vi "Vision Processing.vi"(4 "error in (no error)":errorcluster, 6 "CameraDevRef":T1) -> ()   [LabVIEW 2011]
uses:
  <vilib>/Rock Robotics/WPI/Camera/WPI_CameraDevRef.ctl
  Robot Global Data.vi
  <vilib>/vision/NI_Vision_Development_Module.lvlib
panel:
  in  "Run Calculations":bool
  out "Raw Turret":dbl
  out "Target X Coord":dbl
  out "Target Distance":dbl
  out "Target Y Coord":dbl
  out "Distance Array":dbl[](array[numeric])
  in  "Scaler":dbl=0.85
  in  "Lower Speed Limit":dbl=0.05
  out "Number of Rectangles Visible":dbl
  out "Y Position Array":dbl[](array[numeric])
  out "X Position Array":dbl[](array[numeric])
  in  "View":bool
  out "Target Info":T2(array[cluster])
  in  "Area Size Limit":i32=444
  in  "Particle Count Limit":i32=8
  in  "Score Limits":T3={"Rect Coverage"=76.0, "Aspect Ratio"=40.0, "X Edge Strength"=40.0, "Y Edge Strength"=60.0}
  in  "Processing":enum32{"Color", "Intensity", "Intensity Open"}(tab)=enum."Intensity Open"
  in  "Luminance":i32=255
  in  "Saturation":i32=255
  in  "Hue":i32(knob)=65 scale=0.0..255.0
  in  "Margins":cluster{"Hue":i32, "Sat":i32, "Lum":i32}={"Hue"=20, "Sat"=27, "Lum"=30} {"Sat" scale=0.0..40.0; "Lum" scale=0.0..40.0; "Hue" scale=0.0..40.0}
  in  "Range":cluster{"Lower value":sgl, "Upper value":sgl}={"Lower value"=150.0, "Upper value"=255.0} {"Lower value" scale=0.0..255.0; "Upper value" scale=0.0..255.0}
  in  "Range":cluster{"Lower value":sgl, "Upper value":sgl}={"Lower value"=123.804344, "Upper value"=255.0} {"Lower value" scale=0.0..255.0; "Upper value" scale=0.0..255.0}
  in  "View":bool
  out "Processed Image":T4(plugin-control)
  out "Original Image":T4(plugin-control)
  # "Instructions:\nProcessing the reflective tape that is illuminated by a ring light can be based\non color or light intensity.\nParticles within the image are scored by rectangle coverage, aspect ratio, and\nfor being hollow with a bold edge. A particle is considered a target if all scores\nare above the score limits. Particles can be annotated -- surrounded by\na rectangle and scores drawn to the left .\nTo control the number of particles being scored, use the count limit and the size\nlimit."
  # "To debug, Enable using the View button.\nFor color processing, you can click in the image to select the color for processing."
  # "Enable by clicking the View button.\nGreen scores are above the limit, orange are below. Inner/outer rect\nindicates all passed."
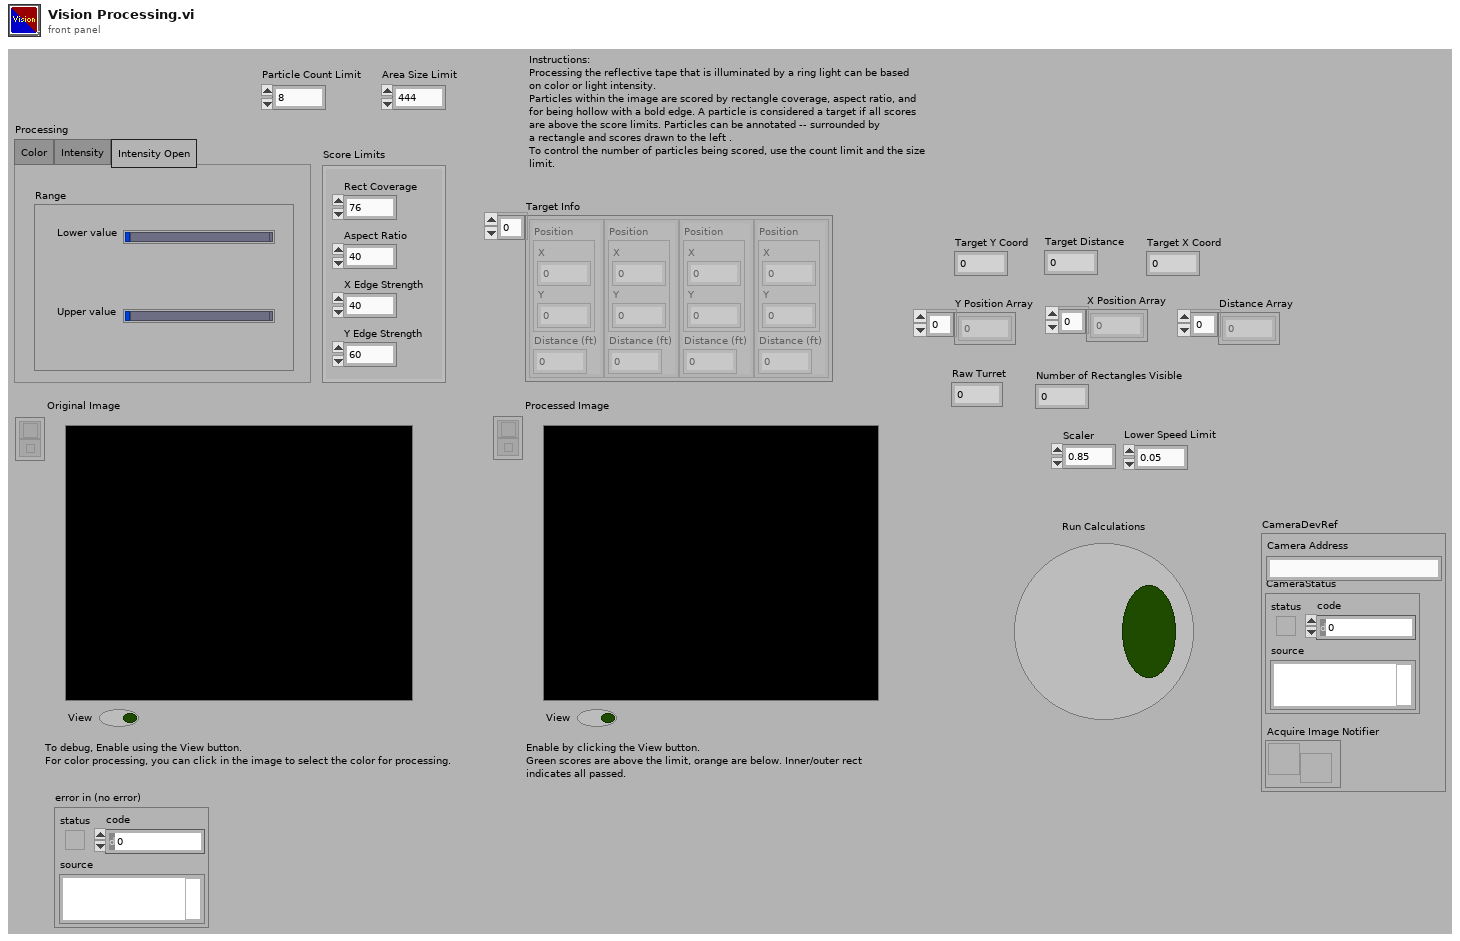
[diagram p1: front panel]
types:
  T1 = typedef "WPI_CameraDevRef.ctl" = cluster{"Camera Address":string, "CameraStatus":errorcluster, "Acquire Image Notifier":refnum<notifier>}
  T2 = cluster{"Position":cluster{"X":dbl, "Y":dbl}, "Distance (ft)":dbl}[]
  T3 = cluster{"Rect Coverage":dbl, "Aspect Ratio":dbl, "X Edge Strength":dbl, "Y Edge Strength":dbl}
  T4 = typedef "IMAQ Image.ctl" = refnum<image>
  T5 = typedef "Image Type" = u32
  T6 = enum32{"AutoM", "Close", "Dilate", "Erode", "Gradient", "Gradient out", "Gradient in", "Hit miss", "Open", "PClose", "POpen", "Thick", "Thin"}
  T7 = typedef "WPI_CameraImageSize.ctl" = enum16{"640x480", "320x240", "160x120"}
  T8 = cluster{"fps":i32, "compression":i32, "Image Size":T7}
  T9 = cluster{cluster{"Left":dbl, "Top":dbl, "Right":dbl, "Bottom":dbl}, dbl[]}[]
  T10 = cluster{"Left":dbl, "Top":dbl, "Right":dbl, "Bottom":dbl}
  T11 = cluster{"Target Center (-1 to 1)":cluster{"X":dbl, "Y":dbl}, "Distance (ft)":dbl}
  T12 = cluster{"Target Center (-1 to 1)":cluster{"X":dbl, "Y":dbl}, "Distance (ft)":dbl}[]
  T13 = typedef "WPI_JoystickDevRef.ctl" = cluster{"Device":T14}
  T14 = typedef "WPI_JoystickDeviceEnum.ctl" = enum16{"USB 1", "USB 2", "USB 3", "USB 4", "Kinect 1", "Kinect 2"}
  T15 = typedef "WPI_JoystickButtonState.ctl" = cluster{"Button 1":bool, "Button 2":bool, "Button 3":bool, "Button 4":bool, "Button 5":bool, "Button 6":bool, "Button 7":bool, "Button 8":bool, "Button 9":bool, "Button 10":bool, "Button 11":bool, "Button 12":bool}
  T16 = cluster{"axis 1 (x)":dbl, "axis 2 (y)":dbl, "axis 3 (throttle)":dbl, "axis 4":dbl, "axis 5":dbl, "axis 6":dbl}
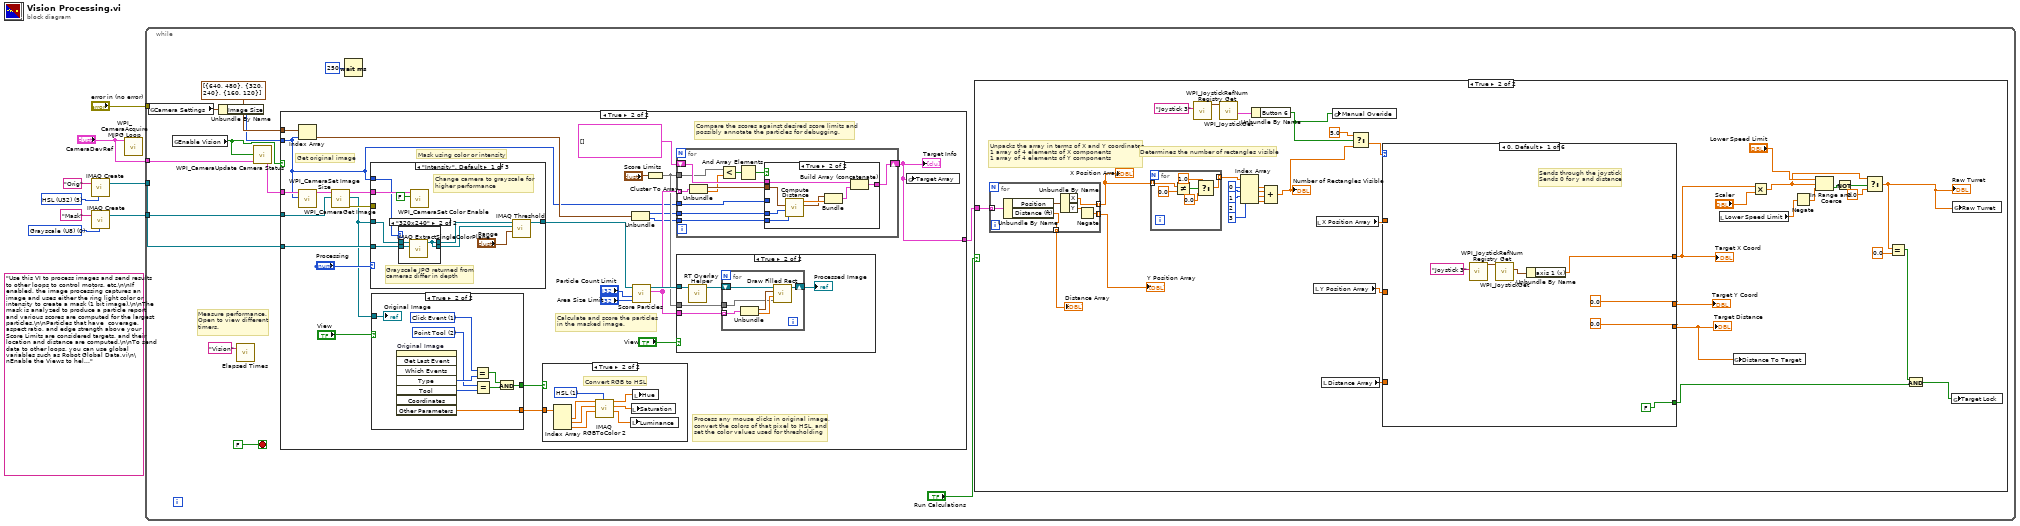
[diagram p0: block diagram]
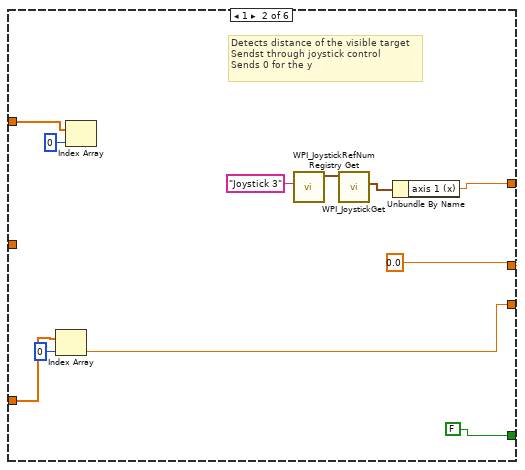
[diagram p3: hidden frame]
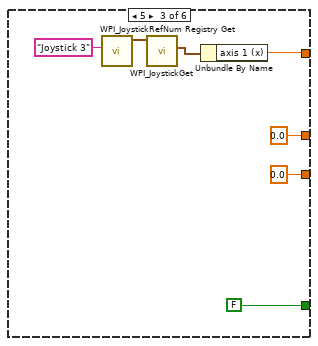
[diagram p4: hidden frame]
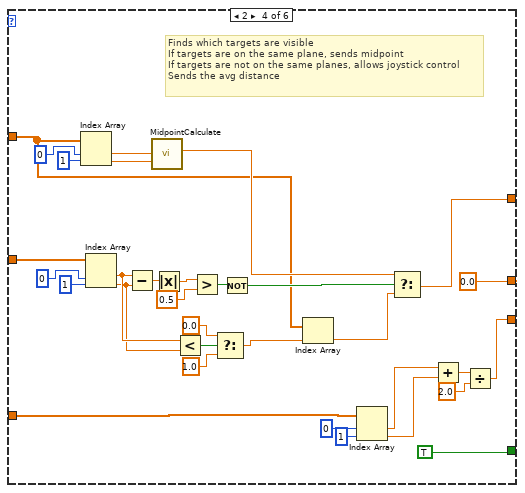
[diagram p5: hidden frame]
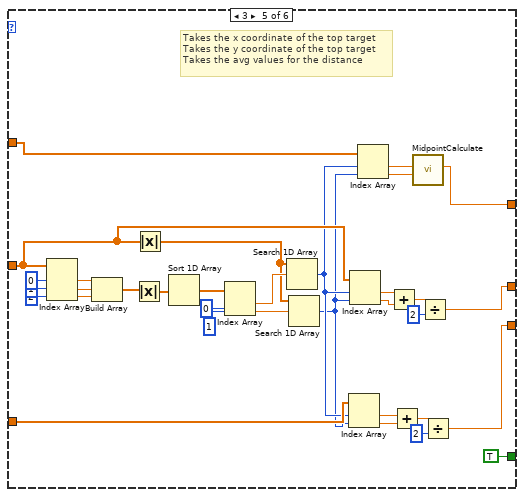
[diagram p6: hidden frame]
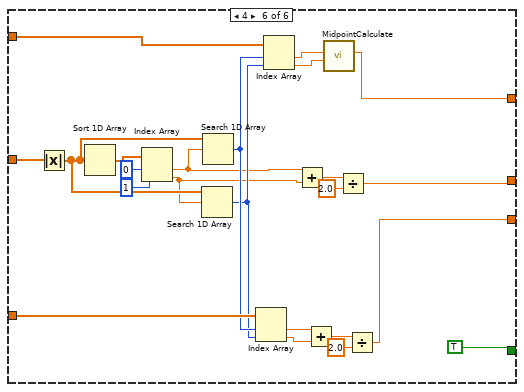
[diagram p7: hidden frame]
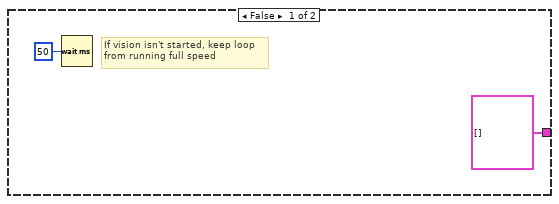
[diagram p8: hidden frame]
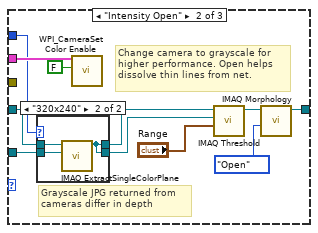
[diagram p11: hidden frame]
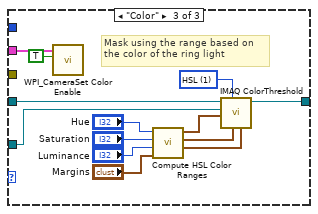
[diagram p13: hidden frame]
diagram:
  w3 = T5 0 items=["Grayscale (U8)", "Grayscale (I16)", "Grayscale (SGL)", "Complex (CSG)", "RGB (U32)", "HSL (U32)", "RGB (U64)", "Grayscale (U16)"] ("Image Type")
  (unwired) "Use this VI to process images and send results to other loops to control motors, etc.\n\nIf enabled, the image processing captures an image and uses either the ring light color or intensity to create a mask (1 bit image).\n\nThe mask is analyzed to produce a particle report and various scores are computed for the largest particles.\n\nParticles that have  coverage, aspect ratio, and edge strength above your Score Limits are considered targets, and their location and distance are computed.\n\nTo send data to other loops, you can use global variables such as Robot Global Data.vi\n\nEnable the Views to help debug color settings. Disable the View to speed up processing."
  w7 = T5 5 items=["Grayscale (U8)", "Grayscale (I16)", "Grayscale (SGL)", "Complex (CSG)", "RGB (U32)", "HSL (U32)", "RGB (U64)", "Grayscale (U16)"] ("Image Type")
  n1 = call "IMAQ Create"("Image Name"="Orig", "Image Type"=w7) -> ("New Image"=w6:T4)  [unwired: 2 in, 2 out]
  n2 = call "IMAQ Create"("Image Name"="Mask", "Image Type"=w3) -> ("New Image"=w1:T4)  [unwired: 2 in, 2 out]
  n3 = call <vilib>:"WPI_CameraAcquire MJPG Loop.vi"("CameraDevRef"="CameraDevRef") -> ()  [unwired: 11 in]
  n4 = while {
    tunnel: w6 -> [w20]
    tunnel: "CameraDevRef" -> [w19]
    tunnel: "error in (no error)" -> [_]
    tunnel: w1 -> [w15]
    stop <- FALSE stop-if-true
    # "Measure performance.\nOpen to view different\ntimers."
    n5 = global read "Robot Global Data.vi" "Camera Settings"() -> (w13:T8)
    n6 = global read "Robot Global Data.vi" "Enable Vision"() -> (w17:bool)
    n7 = Unbundle By Name(w13) -> ("Image Size"=w12:T7)
    n8 = call "Elapsed Times.vi"("Call Name"="Vision") -> ()  [unwired: 2 in, 1 out]
    n9 = call <vilib>:"WPI_CameraUpdate Camera Status.vi"("CameraDevRef In"=w19, "Enable Vision"=w17) -> ("CameraDevRef Out"=w18:T1)  [unwired: 3 in]
    n10 = case shown="True" w17 {
      tunnel: w20 -> [_ w204]
      tunnel: w18 -> [_ w200]
      tunnel: w15 -> [_ w191]
      tunnel: cluster{i32, i32}[] [{640, 480}, {320, 240}, {160, 120}] -> [_ w195]
      tunnel: w12 -> [_ w188]
      tunnel: [T2 [] w189] -> w11
      frame False {
        # "If vision isn't started, keep loop\nfrom running full speed"
        n11 = Wait (ms)(milliseconds to wait=u32 50) -> ()  [unwired: 1 out]
      }
      frame True {
        # "Compare the scores against desired score limits and\npossibly annotate the particles for debugging."
        # "Process any mouse clicks in original image,\nconvert the colors of that pixel to HSL, and\nset the color values used for thresholding"
        # "Calculate and score the particles\nin the masked image."
        # "Mask using color or intensity"
        # "Get original image"
        n12 = call <vilib>:"WPI_CameraSet Image Size.vi"("Image Size"=w188, "CameraDevRef"=w200) -> ("CameraDevRef Out"=w201:T1)  [unwired: 8 in, 1 out]
        n13 = Index Array(array=w195, index=w188) -> (element=w192:cluster{i32, i32})
        n14 = call <vilib>:"WPI_CameraGet Image.vi"("Image"=w204, "CameraDevRef"=w201) -> ("error out"=w202:errorcluster, "Image Out"=w190:T4, "CameraDevRef Out"=w203:T1)  [unwired: 7 in]
        n15 = case shown="\"Intensity\", Default" "Processing" {
          tunnel: w190 -> [w226 w238 w264]
          tunnel: [w229 w243 w263] -> w198
          tunnel: w203 -> [w227 w241 w254]
          tunnel: w202 -> [_ _ _]
          tunnel: w191 -> [w225 w239 w252]
          tunnel: w188 -> [w224 w240 _]
          frame "Intensity", Default {
            # "Grayscale JPG returned from\ncameras differ in depth"
            # "Change camera to grayscale for\nhigher performance"
            n16 = case shown="\"320x240\"" w224 {
              tunnel: w226 -> [w232 w235]
              tunnel: w225 -> [w231 w234]
              tunnel: [w232 w233] -> w223
              tunnel: [w231 w233] -> w222
              frame "640x480", Default {
              }
              frame "320x240" {
                n17 = call "IMAQ ExtractSingleColorPlane"("Image Dst"=w234, "Image Src"=w235) -> ("Image Dst Out"=w233:T4)  [unwired: 8 in, 1 out]
              }
            }
            n18 = call <vilib>:"WPI_CameraSet Color Enable.vi"("Color Enabled"=FALSE, "CameraDevRef"=w227) -> ()  [unwired: 8 in, 2 out]
            n19 = call "IMAQ Threshold"("Range"="Range", "Image Dst"=w222, "Image Src"=w223) -> ("Image Dst Out"=w229:T4)  [unwired: 3 in, 5 out]
          }
          frame "Intensity Open" {
            # "Grayscale JPG returned from\ncameras differ in depth"
            # "Change camera to grayscale for\nhigher performance. Open helps\ndissolve thin lines from net."
            n20 = case shown="\"320x240\"" w240 {
              tunnel: w238 -> [w248 w251]
              tunnel: w239 -> [w247 w250]
              tunnel: [w248 w249] -> w237
              tunnel: [w247 w249] -> w236
              frame "640x480", Default {
              }
              frame "320x240" {
                n21 = call "IMAQ ExtractSingleColorPlane"("Image Dst"=w250, "Image Src"=w251) -> ("Image Dst Out"=w249:T4)  [unwired: 8 in, 1 out]
              }
            }
            n22 = call <vilib>:"WPI_CameraSet Color Enable.vi"("Color Enabled"=FALSE, "CameraDevRef"=w241) -> ()  [unwired: 8 in, 2 out]
            n23 = call "IMAQ Threshold"("Range"="Range", "Image Dst"=w236, "Image Src"=w237) -> ("Image Dst Out"=w244:T4)  [unwired: 3 in, 5 out]
            n24 = call "IMAQ Morphology"("Operation"=T6."Open", "Image Src"=w244) -> ("Image Dst Out"=w243:T4)  [unwired: 8 in, 1 out]
          }
          frame "Color" {
            w262 = u16 1 items=["RGB", "HSL", "HSV", "HSI"] ("Color Mode")
            # "Mask using the range based on\nthe color of the ring light"
            n25 = call <vilib>:"WPI_CameraSet Color Enable.vi"("Color Enabled"=TRUE, "CameraDevRef"=w254) -> ()  [unwired: 8 in, 2 out]
            n26 = call "Compute HSL Color Ranges.vi"("Margins"="Margins", "Luminance"="Luminance", "Saturation"="Saturation", "Hue"="Hue") -> ("Lum Range"=w259:cluster{i32, i32}, "Sat Range"=w260:cluster{i32, i32}, "Hue Range"=w261:cluster{i32, i32})  [unwired: 5 in]
            n27 = call "IMAQ ColorThreshold"("Blue or Luma or Val or Inten Range"=w259, "Green or Sat Range"=w260, "Color Mode"=w262, "Red or Hue Range"=w261, "Image Dst"=w252, "Image Src"=w264) -> ("Image Dst Out"=w263:T4)  [unwired: 4 in, 1 out]
          }
        }
        n28 = case shown="True" "View" {
          tunnel: w190 -> [_ w284]
          tunnel: [_ w279] -> w197
          tunnel: [_ w276] -> w196
          frame False {
          }
          frame True {
            w277 = 2 items=["None", "Selection Tool", "Point Tool", "Line Tool", "Rectangle Tool", "Oval Tool", "Polygon Tool", "ClosedFreehandTool", "Annulus Tool", "Rotated Rectangle Tool", "Zoom Tool", "Pan Tool", "Polyline Tool", "Freehand Tool"] ("Tool")
            w278 = 1 items=["No Event"=0, "Click Event"=1, "Draw Event"=2, "Size Event"=4, "Scroll Event"=5, "Double Click Event"=8] ("Type")
            n29 = invoke on="Original Image" class="ImageControl" method="Get Last Event"() -> ("Type"=w280:i32, "Tool"=w283:i32, "Other Parameters"=w276:sgl[])  [unwired: 8 in, 5 out]
            n30 = Equal?(x=w278, y=w280) -> (x = y?=w281:bool)
            n31 = Equal?(x=w277, y=w283) -> (x = y?=w282:bool)
            n32 = And(x=w281, y=w282) -> (x .and. y?=w279:bool)
            "Original Image" <- w284
          }
        }
        n33 = case shown="True" w197 {
          tunnel: w196 -> [_ w221]
          frame False {
          }
          frame True {
            w220 = u16 1 items=["RGB", "HSL", "HSV", "HSI", "CIE L*a*b*", "CIE XYZ"] ("Color Mode")
            # "Convert RGB to HSL"
            n34 = Index Array(array=w221) -> (element #1=w219:sgl, element #2=w217:sgl, element #3=w215:sgl)  [unwired: 3 in]
            n35 = call "IMAQ RGBToColor 2"("Color Mode"=w220, "Blue value"=w215, "Green value"=w217, "Red value"=w219) -> ("Blue or Luma or Val or Inten or Z or b*value"=w214:dbl, "Green or Sat or Y or a* value"=w216:dbl, "Red or Hue or X or L* value"=w218:dbl)  [unwired: 4 in, 1 out]
            n36 = local write "Luminance"(w214) -> ()
            n37 = local write "Saturation"(w216) -> ()
            n38 = local write "Hue"(w218) -> ()
          }
        }
        n39 = Unbundle(w192) -> (w194:i32, w193:i32)
        n40 = call "Score Particles.vi"("Area Size Limit"="Area Size Limit", "Particle Count Limit"="Particle Count Limit", "Image Refnum in"=w198) -> ("Scored Particle Info"=w209:T9, "Image Refnum out"=w212:T4)  [unwired: 7 in]
        n41 = Cluster To Array(cluster="Score Limits") -> (array=w207:dbl[])
        n42 = for {
          shift-right: [w294] -> w189
          shift-left: T2 [] -> [w295]
          tunnel: w194 -> [w293]
          tunnel: w209 -> [w291] mode=indexing
          tunnel: w207 -> [w286]
          tunnel: w188 -> [w290]
          tunnel: w193 -> [w285]
          n43 = Unbundle(w291) -> (w292:T10, w287:dbl[])
          n44 = Less?(x=w286, y=w287) -> (x < y?=w289:bool[])
          n45 = And Array Elements(Boolean array=w289) -> (logical AND=w288:bool)
          n46 = case shown="True" w288 {
            tunnel: w295 -> [w296 w304]
            tunnel: [w296 w303] -> w294
            tunnel: w292 -> [_ w299]
            tunnel: w293 -> [_ w301]
            tunnel: w290 -> [_ _]
            tunnel: w285 -> [_ w298]
            frame False {
            }
            frame True {
              n47 = call "Compute Distance.vi"("Y Image Resolution"=w298, "X Image Resolution"=w301, "Bounding Box"=w299) -> ("Target Center (-1 to 1)"=w297:cluster{"X":dbl, "Y":dbl}, "Distance (ft)"=w300:dbl)  [unwired: 7 in]
              n48 = Bundle("Target Center (-1 to 1)"=w297, "Distance (ft)"=w300) -> (w302:T11)  [unwired: 1 in]
              n49 = Build Array (concatenate)(w304, w302) -> (w303:T12)
            }
          }
        }
        "Target Info" <- w189
        n50 = case shown="True" "View" {
          tunnel: w212 -> [_ w266]
          tunnel: w209 -> [_ w268]
          tunnel: w207 -> [_ w267]
          frame False {
          }
          frame True {
            n51 = call "RT Overlay Helper.vi"("Refnum in"=w266) -> ("Refnum out"=w269:T4)  [unwired: 10 in]
            n52 = for {
              shift-right: [w274] -> w265
              shift-left: w269 -> [w275]
              tunnel: w268 -> [w271] mode=indexing
              tunnel: w267 -> [w270]
              n53 = Unbundle(w271) -> (w272:T10, w273:dbl[])
              n54 = call "Draw Filled Rect.vi"("Limits"=w270, "Scores"=w273, "Bounding Box"=w272, "image in"=w275) -> ("image out"=w274:T4)  [unwired: 7 in]
            }
            "Processed Image" <- w265
          }
        }
        n55 = global write "Robot Global Data.vi" "Target Array"(w189) -> ()
      }
    }
    n56 = Wait (ms)(milliseconds to wait=u32 250) -> ()  [unwired: 1 out]
    n57 = case shown="True" "Run Calculations" {
      tunnel: w11 -> [_ w33]
      frame False {
      }
      frame True {
        # "Determines the number of rectangles visible"
        # "Unpacks the array in terms of X and Y coordinates\n1 array of 4 elements of X components\n1 array of 4 elements of Y components"
        n58 = for {
          tunnel: [w183] -> w34 mode=indexing
          tunnel: [w184] -> w44 mode=indexing
          tunnel: w33 -> [w181] mode=indexing
          tunnel: [w180] -> w53 mode=indexing
          n59 = Unbundle By Name(w181) -> ("Position"=w185:cluster{"X":dbl, "Y":dbl}, "Distance (ft)"=w180:dbl)
          n60 = Unbundle By Name(w185) -> ("X"=w184:dbl, "Y"=w182:dbl)
          n61 = Negate(x=w182) -> (-x=w183:dbl)
        }
        "X Position Array" <- w44
        "Y Position Array" <- w34
        "Distance Array" <- w53
        n62 = for {
          tunnel: w44 -> [w65] mode=indexing
          tunnel: [w61] -> w43 mode=indexing
          n63 = Not Equal?(x=w65, y=0.0) -> (x != y?=w64:bool)
          n64 = Select(t=1.0, s=w64, f=0.0) -> (s? t:f=w61:dbl)
        }
        n65 = call <vilib>:"WPI_JoystickRefNum Registry Get.vi"("refnum name"="Joystick 3") -> ("JoystickDevRef"=w26:T13)  [unwired: 9 in, 1 out]
        n66 = call <vilib>:"WPI_JoystickGet.vi"("JoystickDevRef"=w26) -> ("Buttons"=w24:T15)  [unwired: 4 in, 2 out]
        n67 = Index Array(array=w43, index #1=0 ("index"), index #2=1 ("index"), index #3=2 ("index"), index #4=3 ("index")) -> (element #1=w41:dbl, element #2=w42:dbl, element #3=w40:dbl, element #4=w39:dbl)
        n68 = Unbundle By Name(w24) -> ("Button 6"=w22:bool)
        n69 = Compound Arithmetic op=ADD(w41, w42, w40, w39) -> (w32:dbl)
        "Number of Rectangles Visible" <- w32
        n70 = local read "Y Position Array"() -> (w56:dbl[])
        n71 = local read "X Position Array"() -> (w45:dbl[])
        n72 = local read "Distance Array"() -> (w57:dbl[])
        n73 = global write "Robot Global Data.vi" "Manual Overide"(w22) -> ()
        n74 = Select(t=5.0, s=w22, f=w32) -> (s? t:f=w59:dbl)
        n75 = case shown="0, Default" w59 {
          tunnel: w45 -> [_ w79 _ w94 w140 w173]
          tunnel: [w67 w74 w85 w112 w137 w163] -> w55
          tunnel: [0.0 ("X") 0.0 ("X") 0.0 ("X") 0.0 ("X") w141 w162] -> w54
          tunnel: [0.0 ("X") w82 0.0 ("X") w105 w125 w157] -> w23
          tunnel: w56 -> [_ _ _ w121 w133 w178]
          tunnel: w57 -> [_ w84 _ w104 w128 w172]
          tunnel: [FALSE FALSE FALSE TRUE TRUE TRUE] -> w29
          frame 0, Default {
            # "Sends through the joystick\nSends 0 for y and distance"
            n76 = call <vilib>:"WPI_JoystickRefNum Registry Get.vi"("refnum name"="Joystick 3") -> ("JoystickDevRef"=w70:T13)  [unwired: 9 in, 1 out]
            n77 = call <vilib>:"WPI_JoystickGet.vi"("JoystickDevRef"=w70) -> ("Axes"=w68:T16)  [unwired: 4 in, 2 out]
            n78 = Unbundle By Name(w68) -> ("axis 1 (x)"=w67:dbl)
          }
          frame 1 {
            # "Detects distance of the visible target\nSendst through joystick control\nSends 0 for the y"
            n79 = Index Array(array=w84, index=0) -> (element=w82:dbl)
            n80 = Index Array(array=w79, index=0) -> ()  [unwired: 1 out]
            n81 = call <vilib>:"WPI_JoystickRefNum Registry Get.vi"("refnum name"="Joystick 3") -> ("JoystickDevRef"=w77:T13)  [unwired: 9 in, 1 out]
            n82 = call <vilib>:"WPI_JoystickGet.vi"("JoystickDevRef"=w77) -> ("Axes"=w75:T16)  [unwired: 4 in, 2 out]
            n83 = Unbundle By Name(w75) -> ("axis 1 (x)"=w74:dbl)
          }
          frame 5 {
            n84 = call <vilib>:"WPI_JoystickRefNum Registry Get.vi"("refnum name"="Joystick 3") -> ("JoystickDevRef"=w88:T13)  [unwired: 9 in, 1 out]
            n85 = call <vilib>:"WPI_JoystickGet.vi"("JoystickDevRef"=w88) -> ("Axes"=w86:T16)  [unwired: 4 in, 2 out]
            n86 = Unbundle By Name(w86) -> ("axis 1 (x)"=w85:dbl)
          }
          frame 2 {
            # "Finds which targets are visible\nIf targets are on the same plane, sends midpoint\nIf targets are not on the same planes, allows joystick control\nSends the avg distance"
            n87 = Index Array(array=w94, index #1=0 ("index"), index #2=1 ("index")) -> (element #1=w110:dbl, element #2=w109:dbl)
            n88 = Index Array(array=w121, index #1=0 ("index"), index #2=1 ("index")) -> (element #1=w100:dbl, element #2=w99:dbl)
            n89 = Subtract(x=w100, y=w99) -> (x-y=w118:dbl)
            n90 = call "MidpointCalculate.vi"("X2"=w109, "X1"=w110) -> ("Midpoint"=w113:dbl)  [unwired: 9 in]
            n91 = Absolute Value(x=w118) -> (abs(x)=w117:dbl)
            n92 = Less?(x=w100, y=w99) -> (x < y?=w98:bool)
            n93 = Greater?(x=w117, y=0.5) -> (0:w114:bool)
            n94 = Select(t=0.0, s=w98, f=1.0) -> (s? t:f=w95:dbl)
            n95 = Not(x=w114) -> (.not. x?=w115:bool)
            n96 = Index Array(array=w94, index=w95) -> (element=w93:dbl)
            n97 = Index Array(array=w104, index #1=0 ("index"), index #2=1 ("index")) -> (element #1=w103:dbl, element #2=w102:dbl)
            n98 = Select(t=w113, s=w115, f=w93) -> (s? t:f=w112:dbl)
            n99 = Add(x=w103, y=w102) -> (x+y=w108:dbl)
            n100 = Divide(x=w108, y=2.0) -> (x/y=w105:dbl)
          }
          frame 3 {
            # "Takes the x coordinate of the top target\nTakes the y coordinate of the top target\nTakes the avg values for the distance"
            n101 = Index Array(array=w133, index #1=0 ("index"), index #2=1 ("index"), index #3=2 ("index")) -> (element #1=w153:dbl, element #2=w152:dbl, element #3=w151:dbl)
            n102 = Build Array(w153, w152, w151) -> (w150:dbl[])
            n103 = Absolute Value(x=w150) -> (abs(x)=w144:dbl[])
            n104 = Absolute Value(x=w133) -> (abs(x)=w136:dbl[])
            n105 = Sort 1D Array(array=w144) -> (sorted array=w149:dbl[])
            n106 = Index Array(array=w149, index #1=0 ("index"), index #2=1 ("index")) -> (element #1=w145:dbl, element #2=w146:dbl)
            n107 = Search 1D Array(1D array=w136, element=w145) -> (index of element=w127:i32)  [unwired: 1 in]
            n108 = Search 1D Array(1D array=w136, element=w146) -> (index of element=w126:i32)  [unwired: 1 in]
            n109 = Index Array(array=w128, index #1=w127, index #2=w126) -> (element #1=w130:dbl, element #2=w129:dbl)
            n110 = Index Array(array=w133, index #1=w127, index #2=w126) -> (element #1=w135:dbl, element #2=w134:dbl)
            n111 = Index Array(array=w140, index #1=w127, index #2=w126) -> (element #1=w139:dbl, element #2=w138:dbl)
            n112 = Add(x=w135, y=w134) -> (x+y=w143:dbl)
            n113 = Add(x=w130, y=w129) -> (x+y=w131:dbl)
            n114 = call "MidpointCalculate.vi"("X2"=w138, "X1"=w139) -> ("Midpoint"=w137:dbl)  [unwired: 9 in]
            n115 = Divide(x=w143, y=2) -> (x/y=w141:dbl)
            n116 = Divide(x=w131, y=2) -> (x/y=w125:dbl)
          }
          frame 4 {
            n117 = Absolute Value(x=w178) -> (abs(x)=w174:dbl[])
            n118 = Sort 1D Array(array=w174) -> (sorted array=w177:dbl[])
            n119 = Index Array(array=w177, index #1=0 ("index"), index #2=1 ("index")) -> (element #1=w169:dbl, element #2=w168:dbl)
            n120 = Search 1D Array(1D array=w174, element=w168) -> (index of element=w170:i32)  [unwired: 1 in]
            n121 = Search 1D Array(1D array=w174, element=w169) -> (index of element=w171:i32)  [unwired: 1 in]
            n122 = Index Array(array=w172, index #1=w171, index #2=w170) -> (element #1=w159:dbl, element #2=w158:dbl)
            n123 = Index Array(array=w173, index #1=w171, index #2=w170) -> (element #1=w165:dbl, element #2=w164:dbl)
            n124 = Add(x=w169, y=w168) -> (x+y=w167:dbl)
            n125 = Add(x=w159, y=w158) -> (x+y=w160:dbl)
            n126 = call "MidpointCalculate.vi"("X2"=w164, "X1"=w165) -> ("Midpoint"=w163:dbl)  [unwired: 9 in]
            n127 = Divide(x=w167, y=2.0) -> (x/y=w162:dbl)
            n128 = Divide(x=w160, y=2.0) -> (x/y=w157:dbl)
          }
        }
        "Target Y Coord" <- w54
        "Target Distance" <- w23
        "Target X Coord" <- w55
        n129 = local read "Lower Speed Limit"() -> (w47:dbl)
        n130 = global write "Robot Global Data.vi" "Distance To Target"(w23) -> ()
        n131 = Multiply(x=w55, y="Scaler") -> (x*y=w52:dbl)
        n132 = Negate(x=w47) -> (-x=w48:dbl)
        n133 = In Range and Coerce(upper limit="Lower Speed Limit", x=w52, lower limit=w48) -> (In Range?=w49:bool)  [unwired: 1 out]
        n134 = Not(x=w49) -> (.not. x?=w50:bool)
        n135 = Select(t=w52, s=w50, f=0.0) -> (s? t:f=w31:dbl)
        "Raw Turret" <- w31
        n136 = Equal?(x=w31, y=0.0) -> (x = y?=w28:bool)
        n137 = And(x=w28, y=w29) -> (x .and. y?=w27:bool)
        n138 = global write "Robot Global Data.vi" "Target Lock"(w27) -> ()
        n139 = global write "Robot Global Data.vi" "Raw Turret"(w31) -> ()
      }
    }
  }
